vi "ReadObjectLayout.vi"(7 "properties to ignore":variant, 8 "error in (no error)":errorcluster, 10 "GObj Refnum":refnum<vi>, 11 "Object Layout in":refnum<class "Object Layout.lvclass">) -> (0 "error out":errorcluster, 3 "Object Layout out":refnum<class "Object Layout.lvclass">)   [LabVIEW 2010, in "NI_SE_Front Panel Layout.lvlib" / "Object Layout.lvclass"]
doc: "Read layout information from the GObj Refnum."
uses:
  Object Layout.lvclass
  Object Layout.lvclass/Object Layout.ctl
  NI_SE_Front Panel Layout.lvlib
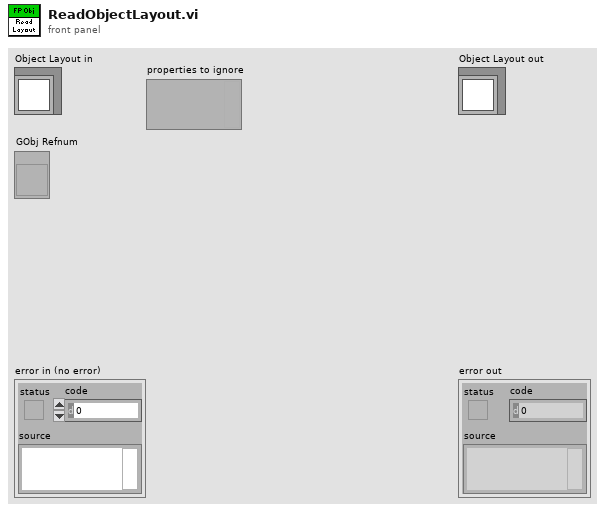
[diagram p1: front panel]
types:
  T1 = typedef "LVRectTypeDef.ctl" = cluster{"left":i16, "top":i16, "right":i16, "bottom":i16}
  T2 = typedef "LVBoundsTypeDef.ctl" = cluster{"Width":u32, "Height":u32}
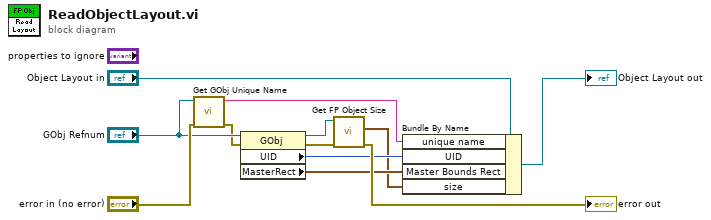
[diagram p0: block diagram]
diagram:
  n1 = call "Get GObj Unique Name.vi"("error in"="error in (no error)", "GObj Refnum"="GObj Refnum") -> ("error out"=w2:errorcluster, "unique name"=w1:string)  [unwired: 7 in, 1 out]
  n2 = property class="GObj"(reference="GObj Refnum", error in=w2) -> (reference out=w5:refnum<vi>, error out=w4:errorcluster, "UID"=w7:i32, "MasterRect"=w6:T1)
  n3 = call "Get FP Object Size.vi"("error in"=w4, "object refnum"=w5) -> ("error out"=→"error out":errorcluster, "size"=w3:T2)  [unwired: 8 in]
  n4 = Bundle By Name(cluster="Object Layout in", "unique name"=w1, "UID"=w7, "Master Bounds Rect"=w6, "size"=w3) -> (→"Object Layout out":refnum<class "Object Layout.lvclass">)
